vi "SysParamByteArr.vi"(9 "idx":u8, 10 "Param Nm":u8) -> (0 "Byte3":u8, 1 "Byte2":u8, 2 "Byte1":u8, 3 "Byte0":u8)   [LabVIEW 2017]
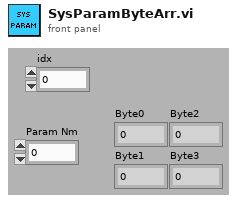
[diagram p1: front panel]
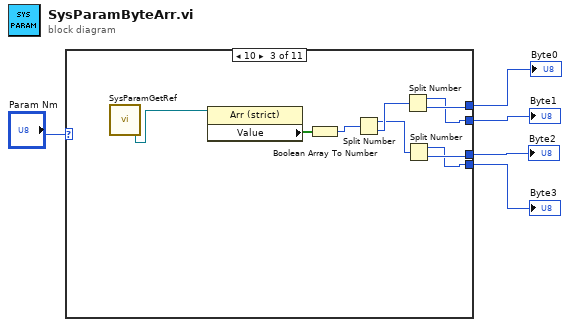
[diagram p0: block diagram]
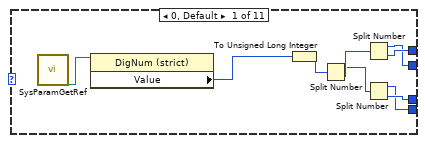
[diagram p2: hidden frame]
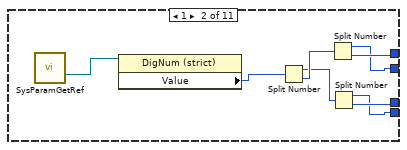
[diagram p3: hidden frame]
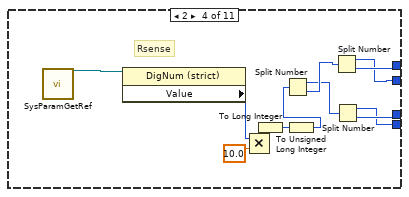
[diagram p4: hidden frame]
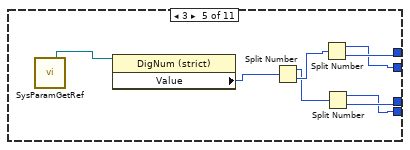
[diagram p5: hidden frame]
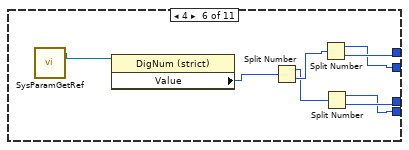
[diagram p6: hidden frame]
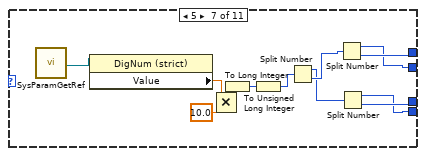
[diagram p7: hidden frame]
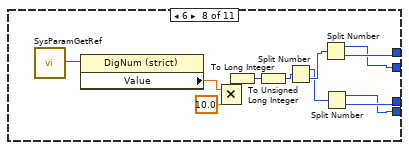
[diagram p8: hidden frame]
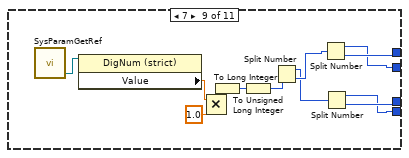
[diagram p9: hidden frame]
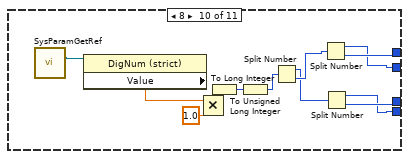
[diagram p10: hidden frame]
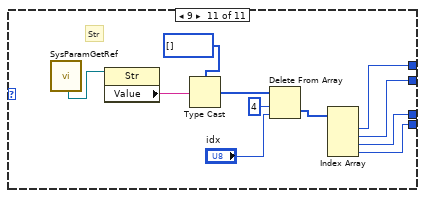
[diagram p11: hidden frame]
diagram:
  n1 = case shown="10" "Param Nm" {
    tunnel: [w12 w19 w29 w41 w48 w56 w69 w81 w93 w105 w111] -> w4
    tunnel: [w11 w18 w28 w40 w47 w55 w68 w80 w92 w104 w110] -> w3
    tunnel: [w10 w17 w27 w39 w46 w54 w67 w79 w91 w103 w109] -> w2
    tunnel: [w9 w16 w26 w38 w45 w53 w66 w78 w90 w102 w108] -> w1
    frame 0, Default {
      n2 = call "SysParamGetRef.vi"() -> ("System Up Time  out"=w6:refnum<vi>)  [unwired: 16 in, 11 out]
      n3 = property class="DigNum (strict)"(reference=w6) -> ("Value"=w7:u32)  [unwired: 1 in, 2 out]
      n4 = To Unsigned Long Integer(number=w7) -> (unsigned 32bit integer=w8:u32)
      n5 = Split Number(x=w8) -> (hi(x)=w13:u16, lo(x)=w14:u16)
      n6 = Split Number(x=w14) -> (hi(x)=w11:u8, lo(x)=w12:u8)
      n7 = Split Number(x=w13) -> (hi(x)=w9:u8, lo(x)=w10:u8)
    }
    frame 1 {
      n8 = call "SysParamGetRef.vi"() -> ("Unit Add out"=w15:refnum<vi>)  [unwired: 16 in, 11 out]
      n9 = property class="DigNum (strict)"(reference=w15) -> ("Value"=w22:u32)  [unwired: 1 in, 2 out]
      n10 = Split Number(x=w22) -> (hi(x)=w20:u16, lo(x)=w21:u16)
      n11 = Split Number(x=w21) -> (hi(x)=w18:u8, lo(x)=w19:u8)
      n12 = Split Number(x=w20) -> (hi(x)=w16:u8, lo(x)=w17:u8)
    }
    frame 10 {
      n13 = call "SysParamGetRef.vi"() -> ("Sys Tech.Data S out"=w25:refnum<vi>)  [unwired: 16 in, 11 out]
      n14 = property class="Arr (strict)"(reference=w25) -> ("Value"=w24:bool[])  [unwired: 1 in, 2 out]
      n15 = Boolean Array To Number(Boolean array=w24) -> (number=w23:u32)
      n16 = Split Number(x=w23) -> (hi(x)=w30:u16, lo(x)=w31:u16)
      n17 = Split Number(x=w31) -> (hi(x)=w28:u8, lo(x)=w29:u8)
      n18 = Split Number(x=w30) -> (hi(x)=w26:u8, lo(x)=w27:u8)
    }
    frame 2 {
      # "Rsense"
      n19 = call "SysParamGetRef.vi"() -> ("R Sense [Ohms] out"=w37:refnum<vi>)  [unwired: 16 in, 11 out]
      n20 = property class="DigNum (strict)"(reference=w37) -> ("Value"=w34:u32)  [unwired: 1 in, 2 out]
      n21 = Multiply(x=w34, y=10.0) -> (x*y=w36:dbl)
      n22 = To Long Integer(number=w36) -> (32bit integer=w35:i32)
      n23 = To Unsigned Long Integer(number=w35) -> (unsigned 32bit integer=w33:u32)
      n24 = Split Number(x=w33) -> (hi(x)=w42:u16, lo(x)=w43:u16)
      n25 = Split Number(x=w43) -> (hi(x)=w40:u8, lo(x)=w41:u8)
      n26 = Split Number(x=w42) -> (hi(x)=w38:u8, lo(x)=w39:u8)
    }
    frame 3 {
      n27 = call "SysParamGetRef.vi"() -> ("Op Amp Gain out"=w44:refnum<vi>)  [unwired: 16 in, 11 out]
      n28 = property class="DigNum (strict)"(reference=w44) -> ("Value"=w51:u32)  [unwired: 1 in, 2 out]
      n29 = Split Number(x=w51) -> (hi(x)=w49:u16, lo(x)=w50:u16)
      n30 = Split Number(x=w50) -> (hi(x)=w47:u8, lo(x)=w48:u8)
      n31 = Split Number(x=w49) -> (hi(x)=w45:u8, lo(x)=w46:u8)
    }
    frame 4 {
      n32 = call "SysParamGetRef.vi"() -> ("RingCancelDelay out"=w52:refnum<vi>)  [unwired: 16 in, 11 out]
      n33 = property class="DigNum (strict)"(reference=w52) -> ("Value"=w59:u32)  [unwired: 1 in, 2 out]
      n34 = Split Number(x=w59) -> (hi(x)=w57:u16, lo(x)=w58:u16)
      n35 = Split Number(x=w58) -> (hi(x)=w55:u8, lo(x)=w56:u8)
      n36 = Split Number(x=w57) -> (hi(x)=w53:u8, lo(x)=w54:u8)
    }
    frame 5 {
      n37 = call "SysParamGetRef.vi"() -> ("Vin Low Th out"=w65:refnum<vi>)  [unwired: 16 in, 11 out]
      n38 = property class="DigNum (strict)"(reference=w65) -> ("Value"=w61:dbl)  [unwired: 1 in, 2 out]
      n39 = Multiply(x=w61, y=10.0) -> (x*y=w63:dbl)
      n40 = To Long Integer(number=w63) -> (32bit integer=w62:i32)
      n41 = To Unsigned Long Integer(number=w62) -> (unsigned 32bit integer=w60:u32)
      n42 = Split Number(x=w60) -> (hi(x)=w70:u16, lo(x)=w71:u16)
      n43 = Split Number(x=w71) -> (hi(x)=w68:u8, lo(x)=w69:u8)
      n44 = Split Number(x=w70) -> (hi(x)=w66:u8, lo(x)=w67:u8)
    }
    frame 6 {
      n45 = call "SysParamGetRef.vi"() -> ("Vin High Th out"=w77:refnum<vi>)  [unwired: 16 in, 11 out]
      n46 = property class="DigNum (strict)"(reference=w77) -> ("Value"=w76:dbl)  [unwired: 1 in, 2 out]
      n47 = Multiply(x=w76, y=10.0) -> (x*y=w74:dbl)
      n48 = To Long Integer(number=w74) -> (32bit integer=w73:i32)
      n49 = To Unsigned Long Integer(number=w73) -> (unsigned 32bit integer=w72:u32)
      n50 = Split Number(x=w72) -> (hi(x)=w82:u16, lo(x)=w83:u16)
      n51 = Split Number(x=w83) -> (hi(x)=w80:u8, lo(x)=w81:u8)
      n52 = Split Number(x=w82) -> (hi(x)=w78:u8, lo(x)=w79:u8)
    }
    frame 7 {
      n53 = call "SysParamGetRef.vi"() -> ("Temp Low Th out"=w89:refnum<vi>)  [unwired: 16 in, 11 out]
      n54 = property class="DigNum (strict)"(reference=w89) -> ("Value"=w85:dbl)  [unwired: 1 in, 2 out]
      n55 = Multiply(x=w85, y=1.0) -> (x*y=w87:dbl)
      n56 = To Long Integer(number=w87) -> (32bit integer=w86:i32)
      n57 = To Unsigned Long Integer(number=w86) -> (unsigned 32bit integer=w84:u32)
      n58 = Split Number(x=w84) -> (hi(x)=w94:u16, lo(x)=w95:u16)
      n59 = Split Number(x=w95) -> (hi(x)=w92:u8, lo(x)=w93:u8)
      n60 = Split Number(x=w94) -> (hi(x)=w90:u8, lo(x)=w91:u8)
    }
    frame 8 {
      n61 = call "SysParamGetRef.vi"() -> ("Temp High Th out"=w101:refnum<vi>)  [unwired: 16 in, 11 out]
      n62 = property class="DigNum (strict)"(reference=w101) -> ("Value"=w97:dbl)  [unwired: 1 in, 2 out]
      n63 = Multiply(x=w97, y=1.0) -> (x*y=w99:dbl)
      n64 = To Long Integer(number=w99) -> (32bit integer=w98:i32)
      n65 = To Unsigned Long Integer(number=w98) -> (unsigned 32bit integer=w96:u32)
      n66 = Split Number(x=w96) -> (hi(x)=w106:u16, lo(x)=w107:u16)
      n67 = Split Number(x=w107) -> (hi(x)=w104:u8, lo(x)=w105:u8)
      n68 = Split Number(x=w106) -> (hi(x)=w102:u8, lo(x)=w103:u8)
    }
    frame 9 {
      # "Str"
      n69 = call "SysParamGetRef.vi"() -> ("System General data out"=w118:refnum<vi>)  [unwired: 16 in, 11 out]
      n70 = property class="Str"(reference=w118) -> ("Value"=w117:string)  [unwired: 1 in, 2 out]
      n71 = Type Cast(type=u8[] [], x=w117) -> (*(type *) &x=w115:u8[])
      n72 = Delete From Array(array=w115, length=4, index="idx") -> (deleted portion=w112:u8[])  [unwired: 1 out]
      n73 = Index Array(array=w112) -> (element #1=w111:u8, element #2=w110:u8, element #3=w109:u8, element #4=w108:u8)  [unwired: 4 in]
    }
  }
  "Byte0" <- w4
  "Byte1" <- w3
  "Byte2" <- w2
  "Byte3" <- w1
